vi "POST_CONSUMO.vi"(0 "DB_API.lvclass":refnum<class "DB_API.lvclass">, 1 "Produccion total":dbl, 2 "Presion baja":dbl, 3 "Presion alta":dbl, 4 "Temperatura":dbl, 5 "Masa baja":dbl, 6 "Masa alta":dbl, 7 "error in (no error)":errorcluster, 13 "Time Stamp":timestamp) -> (20 "DB_API.lvclass 2":refnum<class "DB_API.lvclass">, 22 "body":string, 27 "error out":errorcluster)   [LabVIEW 2024, in "DB_API.lvclass"]
uses:
  DB_API.lvclass
panel:
  out "concatenated string":string
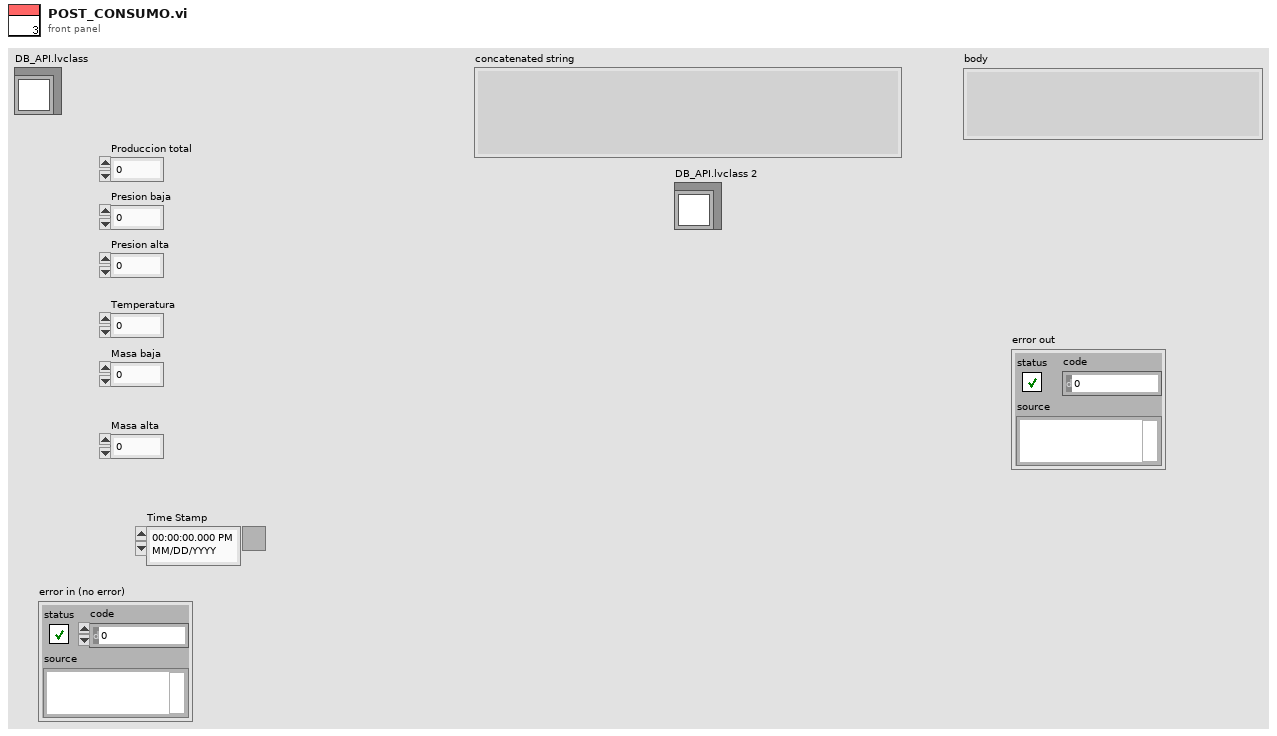
[diagram p1: front panel]
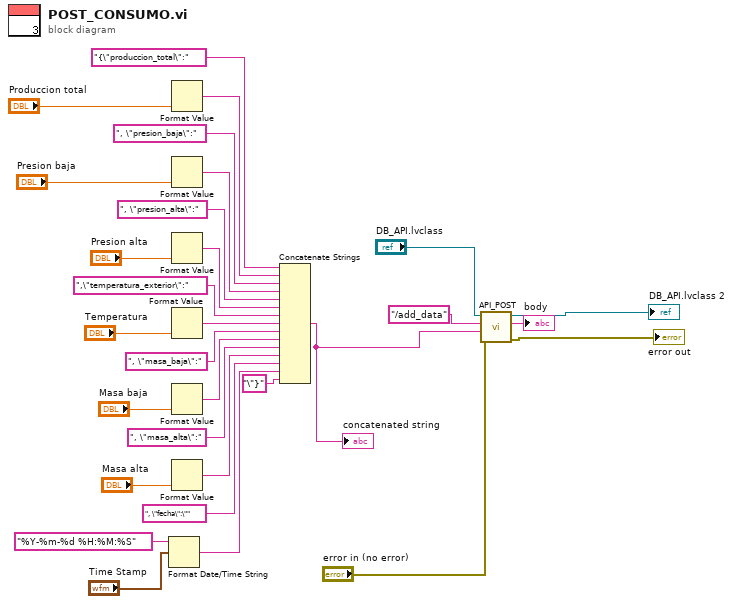
[diagram p0: block diagram]
diagram:
  n1 = Format Date/Time String(time format string (%c)="%Y-%m-%d %H:%M:%S", seconds (now)="Time Stamp") -> (date/time string=w9:string)  [unwired: 1 in]
  n2 = Format Value(value (0)="Produccion total") -> (output string=w23:string)  [unwired: 2 in]
  n3 = Format Value(value (0)="Presion baja") -> (output string=w21:string)  [unwired: 2 in]
  n4 = Format Value(value (0)="Presion alta") -> (output string=w19:string)  [unwired: 2 in]
  n5 = Format Value(value (0)="Temperatura") -> (output string=w17:string)  [unwired: 2 in]
  n6 = Format Value(value (0)="Masa baja") -> (output string=w15:string)  [unwired: 2 in]
  n7 = Format Value(value (0)="Masa alta") -> (output string=w13:string)  [unwired: 2 in]
  n8 = Concatenate Strings("{\"produccion_total\":" ("string"), w23, ", \"presion_baja\":" ("string"), w21, ", \"presion_alta\":" ("string"), w19, ",\"temperatura_exterior\":" ("string"), w17, ", \"masa_baja\":" ("string"), w15, ", \"masa_alta\":" ("string"), w13, ", \"fecha\":\"" ("string"), w9, "\"}" ("string")) -> (w7:string)
  "concatenated string" <- w7
  n9 = call "API_POST.vi"("error in (no error)"="error in (no error)", "buffer"=w7, "endpoint"="/add_data", "DB_API.lvclass"="DB_API.lvclass") -> ("error out"=→"error out":errorcluster, "body"=→"body":string, "output cluster"=→"DB_API.lvclass 2":refnum<class "DB_API.lvclass">)  [unwired: 5 in]
